vi "set_limit.vi"(4 "error in (no error)":errorcluster, 5 "Set Temperature":dbl, 7 "VISA resource name":refnum<visa-resource-name>) -> (0 "error out":errorcluster, 3 "VISA resource name out":refnum<visa-resource-name>)   [LabVIEW 2017]
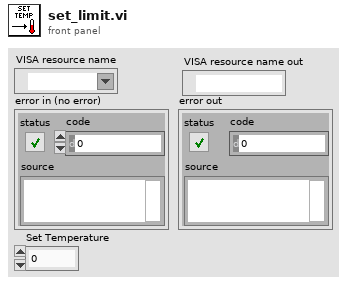
[diagram p1: front panel]
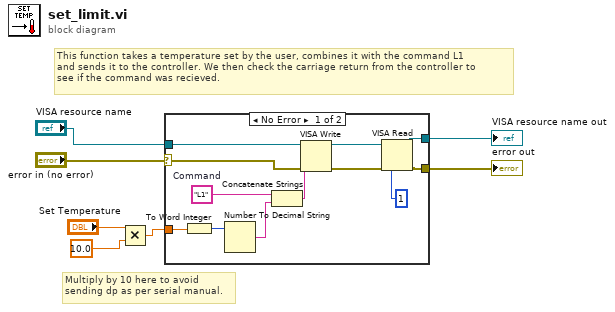
[diagram p0: block diagram]
diagram:
  # "Multiply by 10 here to avoid \nsending dp as per serial manual."
  # "This function takes a temperature set by the user, combines it with the command L1\nand sends it to the controller. We then check the carriage return from the controller to \nsee if the command was recieved."
  n1 = Multiply(x="Set Temperature", y=10.0) -> (x*y=w3:dbl)
  n2 = case shown="No Error" "error in (no error)" {
    selector: "error in (no error)" -> [w17 w20]
    tunnel: "VISA resource name" -> [w18 w21]
    tunnel: w3 -> [w8 _]
    tunnel: [w13 w21] -> w5
    tunnel: [w12 w20] -> w4
    frame No Error {
      w19 = "L1"  # Command
      n3 = To Word Integer(number=w8) -> (16bit integer=w9:i16)
      n4 = Number To Decimal String(number=w9) -> (decimal integer string=w16:string)  [unwired: 1 in]
      n5 = Concatenate Strings(w19, w16) -> (w15:string)
      n6 = VISA Write(VISA resource name=w18, write buffer=w15, error in (no error)=w17) -> (VISA resource name out=w11:refnum<visa-resource-name>, error out=w10:errorcluster)  [unwired: 1 out]
      n7 = VISA Read(VISA resource name=w11, byte count=u32 1, error in (no error)=w10) -> (VISA resource name out=w13:refnum<visa-resource-name>, error out=w12:errorcluster)  [unwired: 2 out]
    }
    frame Error {
    }
  }
  "VISA resource name out" <- w5
  "error out" <- w4
